vi "Create Enqueue Message.vi"(0 "Diagram in":refnum<vi>, 1 "Type":variant, 5 "Inputs":refnum<vi>[](array[refnum]), 11 "error in (no error)":errorcluster, 12 "Cluster":cluster{i32, variant}) -> (4 "Diagram out":refnum<vi>, 10 "error out":refnum<vi>, 15 "error out":errorcluster)   [LabVIEW 2015]
uses:
  source/Scripting.lvlib
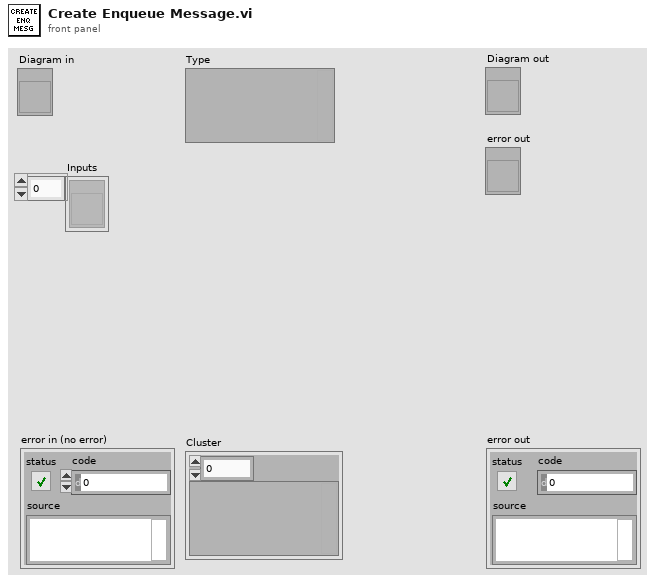
[diagram p1: front panel]
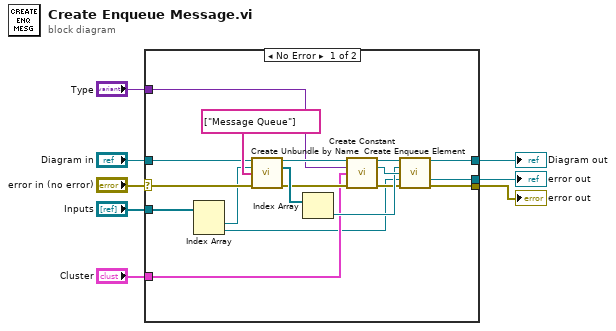
[diagram p0: block diagram]
diagram:
  n1 = case shown="No Error" "error in (no error)" {
    selector: "error in (no error)" -> [w11 w27]
    tunnel: [w26 w27] -> w8
    tunnel: [w25 w28] -> w7
    tunnel: [w24 _] -> w6
    tunnel: "Inputs" -> [w18 _]
    tunnel: "Diagram in" -> [w16 w28]
    tunnel: "Cluster" -> [w14 _]
    tunnel: "Type" -> [w13 _]
    frame No Error {
      n2 = Index Array(array=w18) -> (element #1=w9:refnum<vi>, element #2=w10:refnum<vi>)  [unwired: 2 in]
      n3 = call "Create Unbundle by Name.vi"("Diagram in"=w16, "input cluster"=w9, "Element Names"=string[] ["Message Queue"], "error in (no error)"=w11) -> ("Diagram out"=w17:refnum<vi>, "Outputs"=w21:refnum<vi>[], "error out"=w15:errorcluster)  [unwired: 9 in]
      n4 = Index Array(array=w21) -> (element=w22:refnum<vi>)  [unwired: 1 in]
      n5 = call "Create Constant.vi"("Diagram in"=w17, "Type"=w13, "Value"=w14, "error in (no error)"=w15) -> ("Diagram out"=w20:refnum<vi>, "Terminal"=w23:refnum<vi>, "error out"=w12:errorcluster)  [unwired: 9 in]
      n6 = call "Create Enqueue Element.vi"("Diagram in"=w20, "queue"=w22, "element"=w23, "error in"=w10, "error in (no error)"=w12) -> ("Diagram out"=w25:refnum<vi>, 10:"error out"=w24:refnum<vi>, 15:"error out"=w26:errorcluster)  [unwired: 7 in, 1 out]
    }
    frame Error {
    }
  }
  "error out" <- w8
  "Diagram out" <- w7
  "error out" <- w6
